vi "Packet Decode.vi"(8 "error in (no error)":errorcluster, 10 "Data":u8[](array[numeric]), 11 "Map in":refnum<class "Map.lvclass">) -> (0 "error out":errorcluster, 3 "Map out":refnum<class "Map.lvclass">)   [LabVIEW 2019, in "Map.lvclass"]
uses:
  Map.lvclass
  TCP Packet/Packet.lvclass
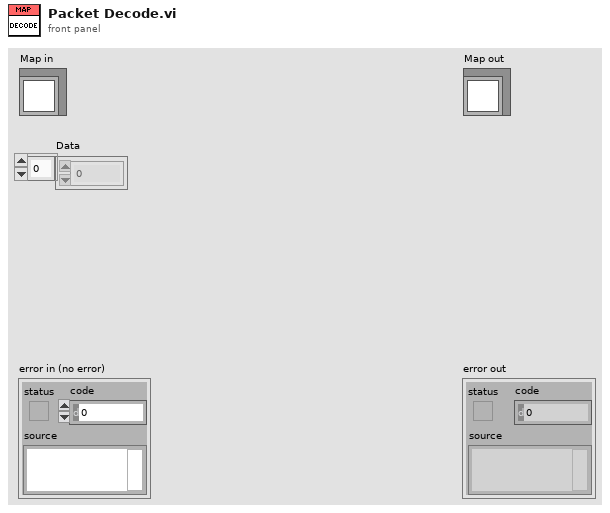
[diagram p1: front panel]
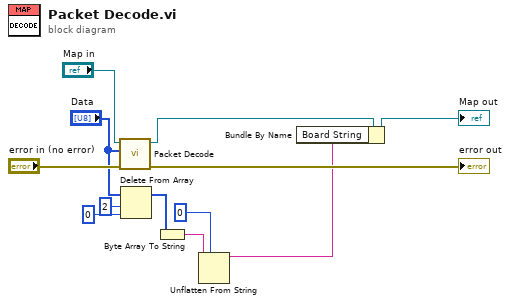
[diagram p0: block diagram]
diagram:
  n1 = call-parent "Packet Decode.vi"("error in (no error)"="error in (no error)", "Data"="Data", "Packet in"="Map in") -> ("error out"=→"error out":errorcluster, "Packet out"=w11:refnum<class "Map.lvclass">)  [unwired: 7 in]
  n2 = Delete From Array(array="Data", length=2, index=0) -> (array with subset deleted=w4:u8[])  [unwired: 1 out]
  n3 = Byte Array To String(unsigned byte array=w4) -> (string=w3:string)
  n4 = Unflatten From String(type=0, binary string=w3) -> (rest of the binary string=w1:string)  [unwired: 3 in, 2 out]
  n5 = Bundle By Name(cluster=w11, "Board String"=w1) -> (→"Map out":refnum<class "Map.lvclass">)
